vi "Multimeter2.vi"(11 "error in":errorcluster) -> (0 "error out":errorcluster, 3 "Voltage":dbl)   [LabVIEW 2017, in "LD Reading.lvclass"]
uses:
  LD Reading.lvclass
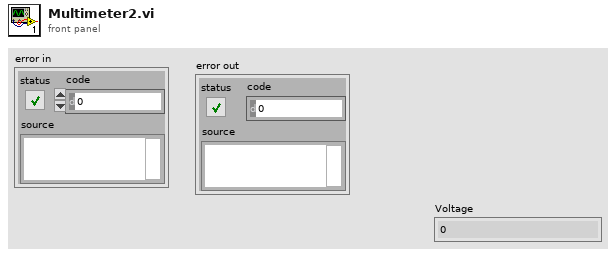
[diagram p1: front panel]
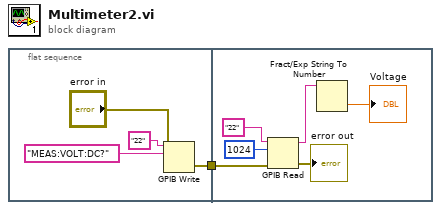
[diagram p0: block diagram]
diagram:
  n1 = flat-sequence {
    tunnel: [w3] -> w1
    tunnel: w1 -> [w11]
    frame #0 {
      n2 = GPIB Write(0:"22" ("address string"), 1:"MEAS:VOLT:DC?" ("data"), 3:"error in") -> (6:w3:errorcluster)  [unwired: 2 in, 1 out]
    }
    frame #1 {
      n3 = GPIB Read(0:"22" ("address string"), 1:1024 ("byte count"), 3:w11) -> (5:w8:string, 7:→"error out":errorcluster)  [unwired: 2 in, 1 out]
      n4 = Fract/Exp String To Number(string=w8) -> (number=→"Voltage":dbl)  [unwired: 3 in, 1 out]
    }
  }
